vi "Run ArduinoCLI.vi"(5 "Console":refnum<vi>, 6 "Python version":string="3.9", 7 "working directory":path=path "/Users/crogers/GitHub/ME35_21/PythonIDE/_LVsubs/Arduino/arduino-cli_0.18.3_macOS_64bit", 8 "error in":errorcluster, 11 "command line":string) -> (0 "error out":errorcluster, 2 "standard output":string, 3 "standard error":string)   [LabVIEW 2022 SP3]
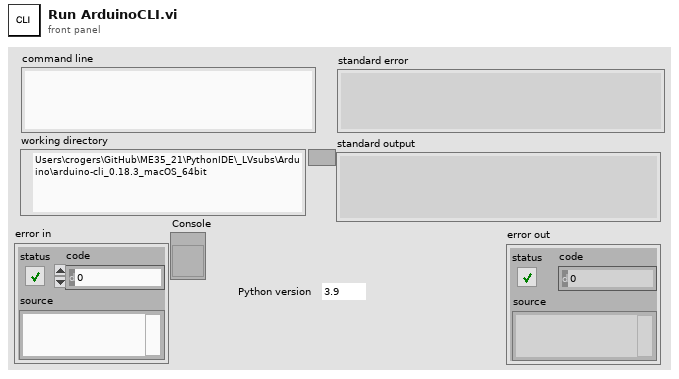
[diagram p1: front panel]
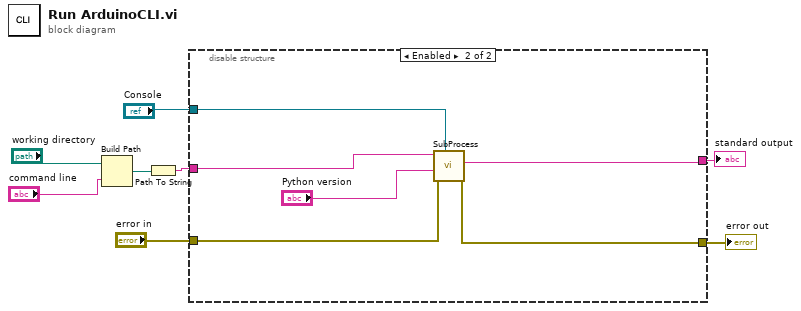
[diagram p0: block diagram]
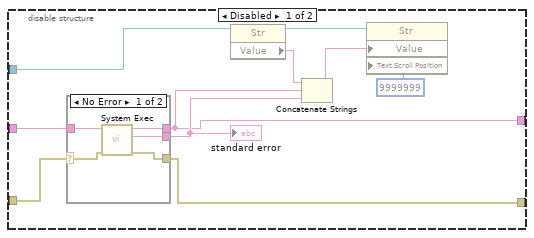
[diagram p2: hidden frame]
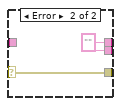
[diagram p3: hidden frame]
diagram:
  n1 = Build Path(base path="working directory", name or relative path="command line") -> (appended path=w7:path)
  n2 = Path To String(path=w7) -> (string=w8:string)
  n3 = disable-structure shown="Enabled" {
    disable-tunnel: w8 -> [w18 w31]
    disable-tunnel: "error in" -> [w17 w27]
    disable-tunnel: "Console" -> [w11 w30]
    disable-tunnel: [w10 w26] -> w2
    disable-tunnel: [w9 w29] -> w1
    frame Disabled {
      n4 = case shown="No Error" w17 {
        selector: w17 -> [w19 w24]
        tunnel: w18 -> [w23 _]
        tunnel: [w22 w25] -> w9
        tunnel: [w20 w24] -> w10
        tunnel: [w21 w25] -> w12
        frame No Error {
          n5 = call <vilib>:"System Exec.vi"("error in (no error)"=w19, "command line"=w23) -> ("error out"=w20:errorcluster, "standard error"=w21:string, "standard output"=w22:string)  [unwired: 6 in, 1 out]
        }
        frame Error {
          w25 = "" ("standard output")
        }
      }
      "standard error" <- w12
      n6 = property class="Str"(reference=w11) -> (reference out=w13:refnum<vi>, "Value"=w15:string)  [unwired: 1 in, 1 out]
      n7 = Concatenate Strings(w15, w9, w12) -> (w14:string)
      n8 = property class="Str"(reference=w13, "Value"=w14, "Text.Scroll Position"=u32 9999999) -> ()  [unwired: 1 in, 2 out]
    }
    frame Enabled {
      n9 = call "SubProcess.vi"("Console"=w30, "error in"=w27, "Python version"="Python version", "Command"=w31) -> ("error out"=w26:errorcluster, "text"=w29:string)  [unwired: 6 in]
    }
  }
  "error out" <- w2
  "standard output" <- w1
